vi "MicroSlideTest.vi"() -> ()   [LabVIEW 2011]
uses:
  <vilib>/Instr/_visa.llb/VISA Configure Serial Port (Instr).vi
panel:
  out "Done!":bool
  in  "Commande":u16(ring) items=["Initialisation", "Mise dans le faisceau", "Retirer du faisceau"]
  in  "send":bool
  out "Received Buffer":string
  out "Active":bool
  in  "quit":bool
  in  "Baud Rate":u32=9600
  in  "VISA resource name":refnum<visa-resource-name>="COM15"
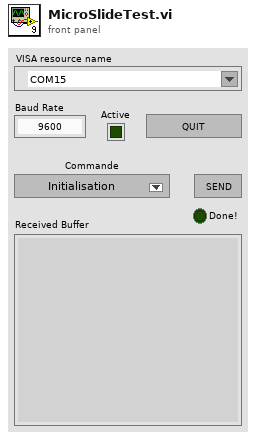
[diagram p1: front panel]
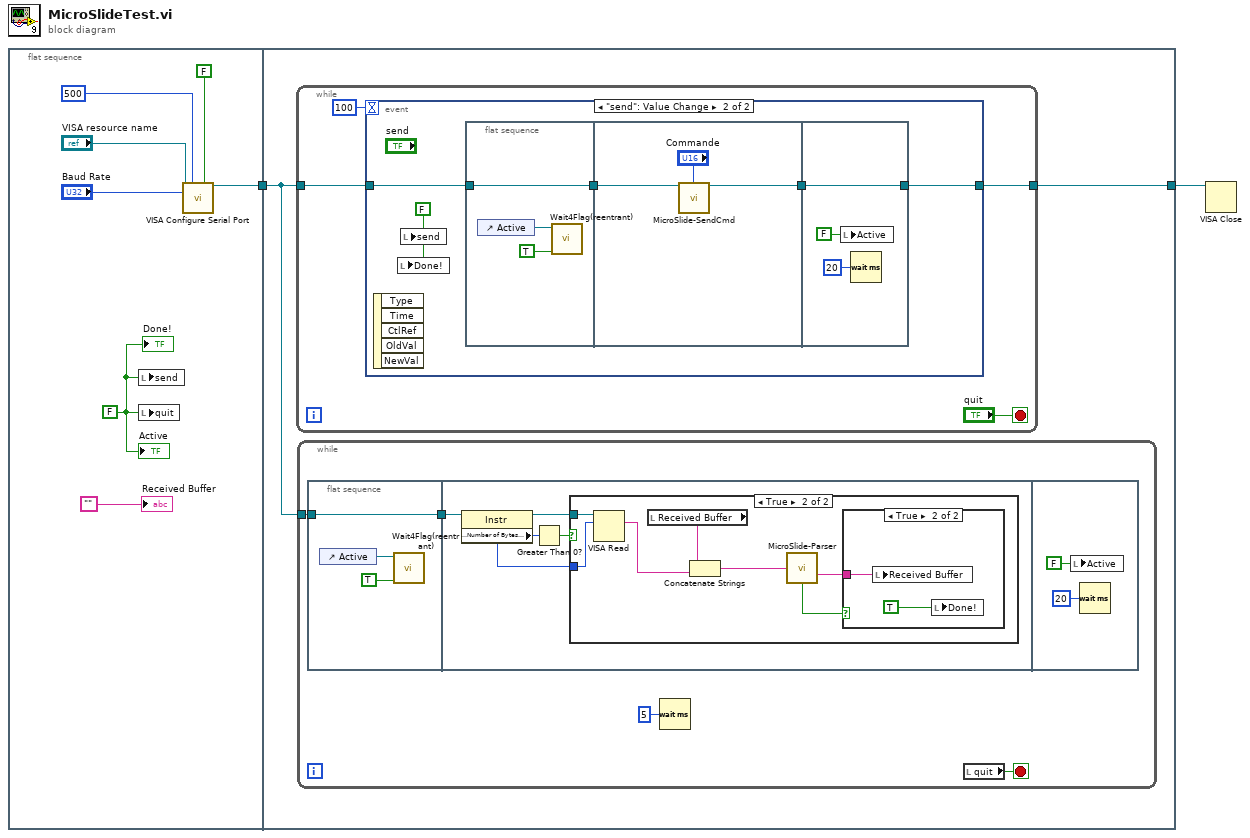
[diagram p0: block diagram]
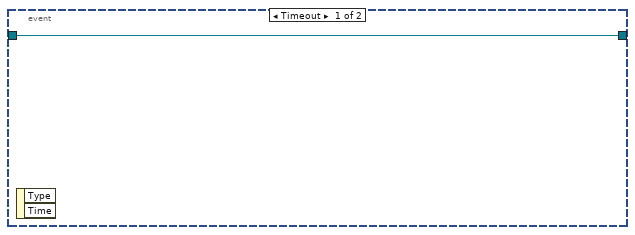
[diagram p2: hidden frame]
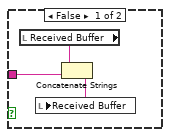
[diagram p4: hidden frame]
diagram:
  n1 = flat-sequence {
    tunnel: [w6] -> w2
    tunnel: w2 -> [w11]
    tunnel: [w10] -> w1
    frame #0 {
      w3 = FALSE ("Enable Termination\nChar (T)")
      n2 = local write "send"(w3) -> ()
      n3 = local write "quit"(w3) -> ()
      n4 = call-poly "VISA Configure Serial Port"("VISA resource name"="VISA resource name", "timeout (10sec)"=u32 500, "Enable Termination\nChar (T)"=FALSE ("Enable Termination\nChar (T)"), "baud rate (9600)"="Baud Rate") -> ("VISA resource name out"=w6:refnum<visa-resource-name>)  [unwired: 10 in, 1 out]
      "Active" <- w3
      "Received Buffer" <- ""
      "Done!" <- w3
    }
    frame #1 {
      n5 = while {
        tunnel: w11 -> [w14]
        tunnel: [w12] -> w10
        stop <- "quit" stop-if-true
        n6 = event shown="[1] \"send\": Value Change" {
          selector: _ -> [_ _]
          dyn-events: _ -> [_ _]
          timeout: 100 -> [_ _]
          tunnel: w14 -> [w16 w20]
          tunnel: [w16 w19] -> w12
          event Timeout {
            n7 = event-data() -> ()  [unwired: 1 in, 2 out]
          }
          event "send": Value Change {
            w17 = FALSE ("send")
            n8 = event-data() -> ()  [unwired: 1 in, 5 out]
            n9 = local write "Done!"(w17) -> ()
            n10 = local write "send"(w17) -> ()
            n11 = flat-sequence {
              tunnel: w20 -> [w24]
              tunnel: [w24] -> w21
              tunnel: w21 -> [w27]
              tunnel: [w26] -> w18
              tunnel: [w28] -> w19
              tunnel: w18 -> [w28]
              frame #0 {
                n12 = control-ref of="Active"() -> (w22:refnum<vi>)
                n13 = call "Wait4Flag(reentrant).vi"("Raise Flag ?"=TRUE, "Ctl Refnum IN"=w22) -> ()  [unwired: 8 in, 2 out]
              }
              frame #1 {
                n14 = call "MicroSlide-SendCmd.vi"("VRN IN"=w27, "Commande"="Commande") -> ("VRN OUT"=w26:refnum<visa-resource-name>)  [unwired: 11 in, 2 out]
              }
              frame #2 {
                n15 = local write "Active"(FALSE ("Active")) -> ()
                n16 = Wait (ms)(milliseconds to wait=u32 20) -> ()  [unwired: 1 out]
              }
            }
          }
        }
      }
      n17 = while {
        tunnel: w11 -> [w33]
        stop <- w34 stop-if-true
        n18 = flat-sequence {
          tunnel: w33 -> [w37]
          tunnel: [w37] -> w32
          tunnel: w32 -> [w41]
          frame #0 {
            n19 = control-ref of="Active"() -> (w35:refnum<vi>)
            n20 = call "Wait4Flag(reentrant).vi"("Raise Flag ?"=TRUE, "Ctl Refnum IN"=w35) -> ()  [unwired: 8 in, 2 out]
          }
          frame #1 {
            n21 = property class="Instr"(reference=w41) -> (reference out=w39:refnum<visa-resource-name>, "Serial Settings:Number of Bytes at Serial Port"=w38:u32)  [unwired: 1 in, 1 out]
            n22 = Greater Than 0?(x=w38) -> (x > 0?=w40:bool)
            n23 = case shown="True" w40 {
              tunnel: w39 -> [_ w48]
              tunnel: w38 -> [_ w47]
              frame False {
              }
              frame True {
                n24 = VISA Read(VISA resource name=w48, byte count=w47) -> (read buffer=w43:string)  [unwired: 1 in, 3 out]
                n25 = local read "Received Buffer"() -> (w44:string)
                n26 = Concatenate Strings(w44, w43) -> (w42:string)
                n27 = call "MicroSlide-Parser.vi"("String"=w42) -> ("Leftovers"=w45:string, "Received"=w46:bool)  [unwired: 12 in, 1 out]
                n28 = case shown="True" w46 {
                  tunnel: w45 -> [w49 w52]
                  frame False {
                    n29 = local read "Received Buffer"() -> (w51:string)
                    n30 = Concatenate Strings(w51, w49) -> (w50:string)
                    n31 = local write "Received Buffer"(w50) -> ()
                  }
                  frame True {
                    n32 = local write "Received Buffer"(w52) -> ()
                    n33 = local write "Done!"(TRUE ("Done!")) -> ()
                  }
                }
              }
            }
          }
          frame #2 {
            n34 = local write "Active"(FALSE ("Active")) -> ()
            n35 = Wait (ms)(milliseconds to wait=u32 20) -> ()  [unwired: 1 out]
          }
        }
        n36 = Wait (ms)(milliseconds to wait=u32 5) -> ()  [unwired: 1 out]
        n37 = local read "quit"() -> (w34:bool)
      }
    }
  }
  n38 = VISA Close(VISA resource name=w1) -> ()  [unwired: 1 in, 1 out]
